vi "txttest.vi"() -> ()   [LabVIEW 2016, in "数据传输系统-02.lvlib" / "自动更新.lvlib" / "TCP文件传输系统.lvlib"]
uses:
  <vilib>/Utility/sysdir.llb/System Directory Type.ctl
panel:
  out "TCP发送全局簇":T1
  out "文件传输的路径":path
  in  "Application":string="版本升级文档.txt"
  in  "远程端口或服务名称":u16=11235
  out "本机网络地址":string="192.168.1.250"
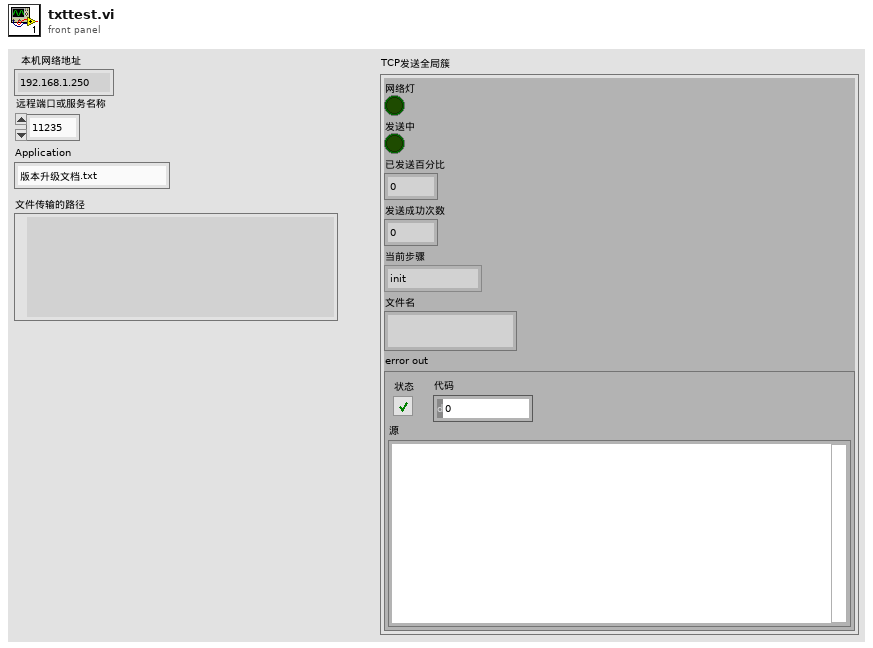
[diagram p1: front panel]
types:
  T1 = cluster{"网络灯":bool, "发送中":bool, "已发送百分比":u8, "发送成功次数":dbl, "当前步骤":enum16{"init", "sendhead", "sendcontent", "sendsuccess", "over"}, "文件名":string, "error out":errorcluster}
  T2 = typedef "System Directory Type.ctl" = i32
  T3 = cluster{"网络灯":bool, "发送中":bool, "已发送百分比":u8, "发送成功次数":dbl, "当前步骤":enum16{"readfile", "init", "sendhead", "sendcontent", "sendsuccess", "over"}, "文件名":string, "error out":errorcluster}
  T4 = enum32{"Bad", "Idle", "Run top level", "Running"}
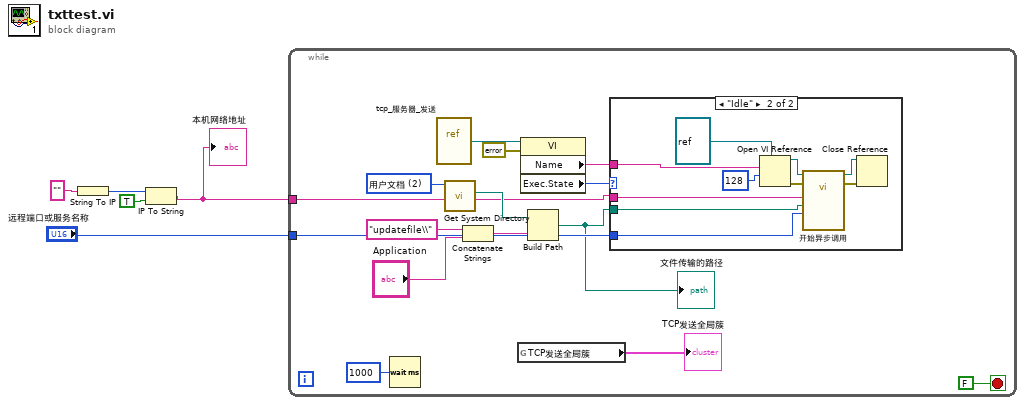
[diagram p0: block diagram]
diagram:
  n1 = String To IP(1:"" ("名称")) -> (0:w3:u32)
  n2 = IP To String(1:TRUE ("句点符号？(F)"), 2:w3) -> (0:w1:string)
  "本机网络地址" <- w1
  n3 = while {
    tunnel: w1 -> [w11]
    tunnel: "远程端口或服务名称" -> [w10]
    stop <- FALSE stop-if-true
    w15 = T2 2 items=["用户目录"=0, "用户桌面"=1, "用户文档"=2, "用户应用程序数据"=3, "用户设置"=4, "用户临时目录"=5, "公共文档"=6, "公共应用程序数据"=7, "公共设置"=8, "公共缓存"=13, "系统核心库"=9, "系统安装库"=10, "应用程序文件"=11, "启动盘根目录"=12] ("system directory type")
    n4 = Wait (ms)(milliseconds to wait=u32 1000 ("等待时间（毫秒）")) -> ()  [unwired: 1 out]
    n5 = vi-ref "tcp_服务器_发送.vi"() -> (w14:refnum<vi>)
    n6 = call <vilib>:"Get System Directory.vi"("system directory type"=w15) -> ("system directory"=w16:path)  [unwired: 10 in]
    n7 = Concatenate Strings("updatefile\\" ("condition"), "Application") -> (w18:string)
    n8 = global read "全局变量1.vi" "TCP发送全局簇"() -> (→"TCP发送全局簇":T3)
    n9 = property class="VI"(reference=w14, error in=errorcluster {"status"=FALSE, "code"=0, "source"=""} ("错误输出")) -> ("Name"=w13:string, "Exec.State"=w19:T4)  [unwired: 2 out]
    n10 = Build Path(base path=w16, name or relative path=w18) -> (appended path=w9:path)
    "文件传输的路径" <- w9
    n11 = case shown="\"Idle\"" w19 {
      tunnel: w13 -> [_ w30]
      tunnel: w11 -> [_ w23]
      tunnel: w9 -> [_ w22]
      tunnel: w10 -> [_ w21]
      frame "Bad", Default {
      }
      frame "Idle" {
        n12 = Open VI Reference(type specifier VI Refnum (for type only)=refnum<vi> refnum, vi path=w30, options=128 ("选项")) -> (vi reference=w28:refnum<vi>, error out=w26:errorcluster)  [unwired: 3 in]
        n13 = call-by-ref "开始异步调用"(reference=w28, error in=w26, "远程端口或服务名称"=w21, "原文件路径（使用对话框）"=w22, "服务器网络地址"=w23) -> (reference out=w24:refnum<vi>, error out=w25:errorcluster)  [unwired: 9 in]
        n14 = Close Reference(reference=w24, error in (no error)=w25) -> ()  [unwired: 1 out]
      }
    }
  }
